vi "Air Heater Control System Example.vi"() -> ()   [LabVIEW 2017]
uses:
  <vilib>/Simulation/Scripting/Companion Diagram/SimConfigNode/SimParams.ctl
  <vilib>/Simulation/Scripting/Companion Diagram/SimConfigNode/_simSolvers.ctl
  <vilib>/Simulation/Implementation/Shared/SIMSCR Execution Mode.ctl
  <vilib>/Simulation/Param Hierarchy/Typedefs/SIMPH Param Control Actions.ctl
  <vilib>/Simulation/Implementation/Shared/NILVSim_ParamChanged.vi
  <vilib>/Simulation/Implementation/Shared/NILVSIM_BeginStep.vi
  <vilib>/Simulation/Implementation/Shared/NILVSim_Manager.vi
  <vilib>/Utility/error.llb/Clear Errors.vi
  <vilib>/Simulation/Implementation/Shared/NILVSim_FinalizeModel.vi
  <vilib>/Simulation/Implementation/Shared/SIM Unbundle Sim Info.vi
  <vilib>/Simulation/Implementation/Shared/NILVSim_Initialize.vi
  <vilib>/Simulation/Utility/Implementation/NILVSim Get Time and IsAcceptedStep.vi
  <vilib>/Simulation/Implementation/Shared/SIMSH Read Queue.vi
  <vilib>/Simulation/Implementation/Shared/NILVSim_GetModelError.vi
  <vilib>/Simulation/Implementation/Shared/SIM Bundle Sim Info.vi
  <vilib>/Simulation/Implementation/XNodeFramework/SimXNode/SimX.xnode
  Air Heater Black Box Model.vi
  <vilib>/Simulation/Scripting/Companion Diagram/SimConfigNode/SimDog.xnode
  <vilib>/Simulation/Implementation/Shared/NI_SIM_Implementation.lvlib
panel:
  out "Control Chart":dbl(graph)=1.1724378087907898
  out "Measurement Chart":dbl(graph)
  in  "Stop":bool
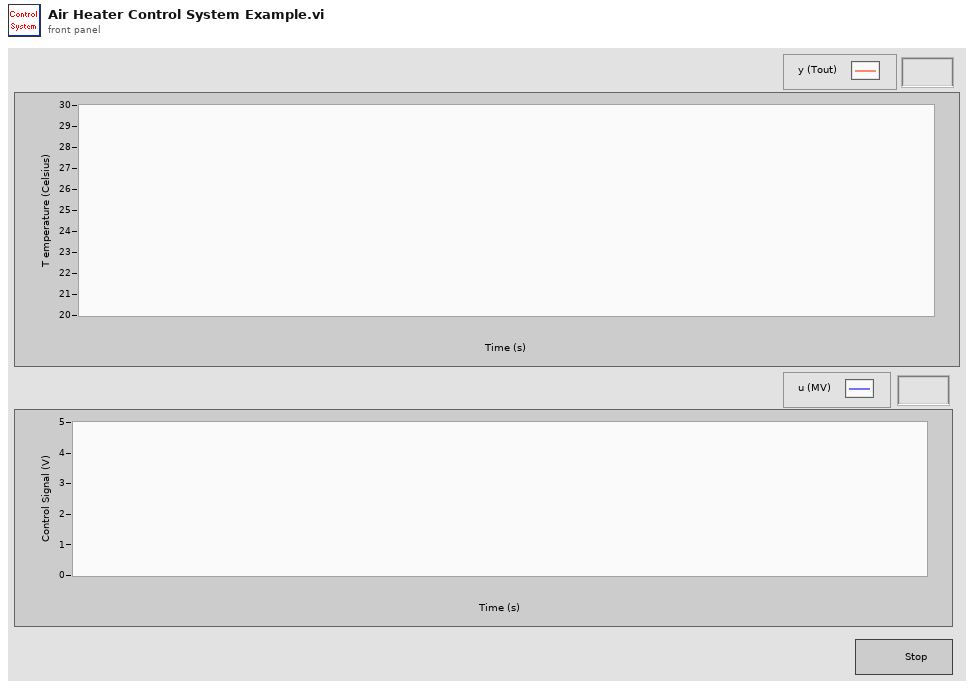
[diagram p1: front panel]
types:
  T1 = enum16{"Simulate to Completion", "Single Time-Step Simulation (Fixed Step Only)"}
  T2 = typedef "SIMSCR Execution Mode.ctl" = enum16{"Simulate to Completion", "Single Time-Step Simulation (Fixed Step Only)"}
  T3 = typedef "SIMPH Param Control Actions.ctl" = enum16{"get params", "set params"}
  T4 = cluster{"SIMSH Sim Time":dbl, "Select":cluster{"s? t:f":dbl}, "Linear Scaling with Points.vi":cluster{"y":dbl}, "Summation 3":cluster{"Result":dbl}, "Square Root":cluster{"sqrt(x)":dbl}, "Gaussian White Noise PtByPt.vi":cluster{"Gaussian white noise":dbl}, "Integrator":cluster{"output":dbl}, "Multiplication":cluster{"Result":dbl}, "Summation":cluster{"Result":dbl}, "Multiplication 2":cluster{"Result":dbl}, "Transport Delay":cluster{"output":dbl}, "Summation 2":cluster{"Result":dbl}}
  T5 = typedef "SimParams.ctl" = cluster{"Initial Time (s)":dbl, "Final Time (s)":dbl, "Step Size (s)":dbl, "ODE Solver":T6, "Minimum Step Size (s)":dbl, "Maximum Step Size (s)":dbl, "Relative Tolerance":dbl, "Absolute Tolerance":dbl, "Software Timing":bool, "Initial Step Size (s)":dbl, "Automatic Fixed Step Size?":bool, "Automatic Discrete Step Size?":bool, "Discrete Step Size (s)":dbl, "Calculate using Time Step":bool, "Solver Wired?":bool, "Prev.Frm.Expected End":u64, "Prev.Frm.Actual End":u64, "Prev.Frm.Finished Late?":bool, "Prev.Iter.Expected End":u64, "Prev.Iter.Actual End":u64, "Prev.Iter.Finished Late?":bool, "Expected Iteration Start":u64, "Actual Iteration Start":u64, "Expected Frame Start":u64, "Actual Frame Start":u64, "Source Name":string, "Name":string, "Period":i64, "Deadline":i64, "Offset":i64, "Start":i64, "Priority":i32, "Timeout":i32, "Processor":i32, "Mode":enum32{"No Change", "Process missed periods, maintain original phase", "Discard missed periods, maintain original phase", "Process missed periods, ignore original phase", "Discard missed periods, ignore original phase"}, "Wakeup reason":enum32{"Normal", "Aborted", "Asynchronous wakeup", "Timing source error", "Timed loop error", "Timeout"}, "Error":errorcluster, "Source Type":string, "Secondary Source Type":string, "Global End Time":u64, "Global Start Time":u64, "Full Solver Reset":bool, "Execution Mode":T2, "Nan/Inf Check":bool, "Custom Solver Library":string, "Solver Is Variable":bool, "custom solver name":string, "Signal Collection Decimation":u32}
  T6 = typedef "_simSolvers.ctl" = enum16{"Runge-Kutta 1 (Euler)", "Runge-Kutta 2", "Runge-Kutta 3", "Runge-Kutta 4", "Runge-Kutta 23 (variable)", "Runge-Kutta 45 (variable)", "BDF (variable)", "Adams-Moulton (variable)", "Rosenbrock (variable)", "Discrete States Only", "SDIRK 4 (variable)", "Radau 5 (variable)", "Radau 9 (variable)", "Radau 13 (variable)", "Radau [Variable Order] (variable)", "Gear's Method (variable)", "Linearizer", "State Query", "Trim Eval", "Custom Solver"}
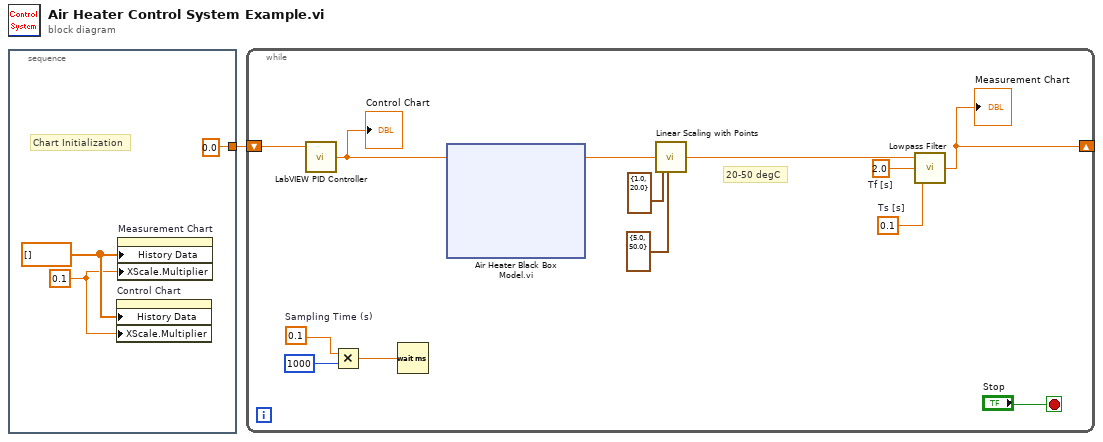
[diagram p0: block diagram]
diagram:
  n1 = stacked-sequence {
    tunnel: [0.0 ("Tout")] -> w1
    frame #0 {
      w2 = 0.1 ("X Scale.Offset and Multiplier:Multiplier")
      w3 = dbl[] [] ("History Data")
      # "Chart Initialization"
      n2 = property on="Control Chart" class="WFChart (strict)"("History Data"=w3, "XScale.Multiplier"=w2) -> ()  [unwired: 2 in, 2 out]
      n3 = property on="Measurement Chart" class="WFChart (strict)"("History Data"=w3, "XScale.Multiplier"=w2) -> ()  [unwired: 2 in, 2 out]
    }
  }
  n4 = while {
    shift-right: [w5] -> _
    shift-left: w1 -> [w11]
    stop <- "Stop" stop-if-true
    w9 = 0.1  # Ts [s]
    w8 = 2.0  # Tf [s]
    w14 = 0.1  # Sampling Time (s)
    # "20-50 degC"
    n5 = call "LabVIEW PID Controller.vi"("Process Variable"=w11) -> ("Control Value"=w10:dbl)  [unwired: 2 in]
    "Control Chart" <- w10
    n6 = Multiply(x=w14, y=1000) -> (x*y=w16:dbl)
    n7 = Wait (ms)(milliseconds to wait=w16) -> ()  [unwired: 1 out]
    n8 = xnode "Air Heater Black Box Model.vi"("Control Signal [0-5V]"=w10) -> ("Tout [1-5V]"=w7:dbl)  [unwired: 2 in, 1 out]
    n9 = call "Linear Scaling with Points.vi"("x"=w7, "Point1"=cluster{"x1":dbl, "y1":dbl} {"x1"=1.0, "y1"=20.0}, "Point2"=cluster{"x2":dbl, "y2":dbl} {"x2"=5.0, "y2"=50.0}) -> ("y"=w6:dbl)  [unwired: 12 in]
    n10 = call "Lowpass Filter.vi"("Ts [s]"=w9, "Tf [s]"=w8, "Filter Input"=w6) -> ("Filter Output"=w5:dbl)
    "Measurement Chart" <- w5
  }
